vi "Configure PointScan.vi"(0 "AODAcq in":refnum<class "AODAcq.lvclass">, 3 "Recording Settings":T1, 5 "Points":i32[][](array[numeric]), 7 "GridSize":u32, 9 "Reps":u32, 11 "error in (no error)":errorcluster, 12 "Motion Points":u32, 14 "Motion Increment":u32) -> (4 "AODAcq out":refnum<class "AODAcq.lvclass">, 15 "error out":errorcluster)   [LabVIEW 2011, in "AODAcq.lvclass"]
uses:
  AODAcq.lvclass
  AODAcq.lvclass/AODAcq.ctl
  <vilib>/Utility/error.llb/Error Cluster From Error Code.vi
  Program Files/National Instruments/LabVIEW 2011/Targets/NI/FPGA/StockFPGA_IntfPrivate/ScriptTemplates/StockFPGA_PlugInRead32.vi
  <vilib>/rvi/errors/niLvFpgaAdjustHostInterfaceError.vi
  <instrlib>/niHWS/nihws.llb/niHWS Write Analog I32.vi
  <vilib>/rvi/interface/nirviReadWriteControl/nirviReadWriteControl.xnode
  FPGA_Control/AODRef.ctl
  FPGA_Control/FPGA Bitfiles/AODControl_FPGATarget_5751Acquire_F1CF9257.lvbitx
  FPGA_Control/AOD Control (FPGA).vi
  NiFpgaLv.dll
  <vilib>/FPGAPlugInAG/PXIe-7965R/niLvFpga_Read32_PXIe-7965R.vi
  <vilib>/rvi/interface/nirviReadWriteControl/niFpgaRWControlAccessTimeoutTemplate.vi
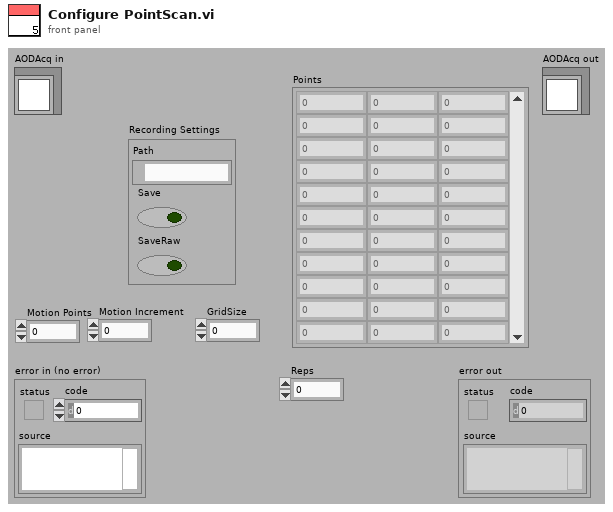
[diagram p1: front panel]
types:
  T1 = cluster{"Path":path, "Save":bool, "SaveRaw":bool}
  T2 = typedef "AODRef.ctl" = refnum<k20>
  T3 = cluster{"file handle out":u32, "ImData":u32[], "TemporalData":u32[], "MotionData":u32[], "stream reference":u32, "Open":bool, "RecordRaw":bool}
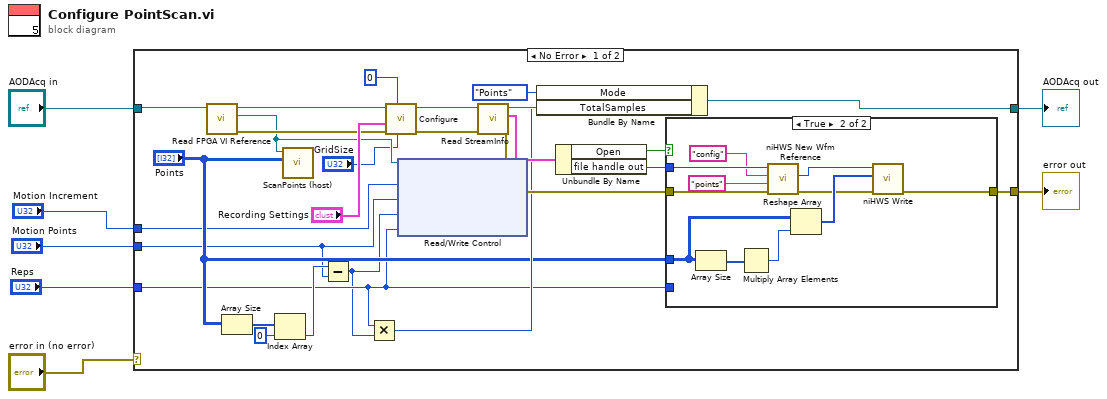
[diagram p0: block diagram]
diagram:
  n1 = case shown="No Error" "error in (no error)" {
    selector: "error in (no error)" -> [_ w47]
    tunnel: [w22 w47] -> w6
    tunnel: [w18 w46] -> w4
    tunnel: "AODAcq in" -> [w31 w46]
    tunnel: "Motion Increment" -> [w13 _]
    tunnel: "Motion Points" -> [w11 _]
    tunnel: "Reps" -> [w10 _]
    frame No Error {
      n2 = call-dynamic "Read FPGA VI Reference.vi"("AODAcq in"=w31) -> ("error out"=w28:errorcluster, "FPGA VI Reference"=w14:T2, "AODAcq out"=w30:refnum<class "AODAcq.lvclass">)  [unwired: 8 in]
      n3 = Array Size(array="Points") -> (size(s)=w21:i32[])
      n4 = Index Array(array=w21, index=0) -> (element=w12:i32)
      n5 = call "ScanPoints (host).vi"("Points"="Points", "FPGA VI Reference Out"=w14) -> ()  [unwired: 10 in]
      n6 = Subtract(x=w12, y=w11) -> (x-y=w9:u32)
      n7 = Multiply(x=w10, y=w9) -> (x*y=w17:u32)
      n8 = call-dynamic "Configure.vi"("GridSize"="GridSize", "Mode"=u32 0, "error in (no error)"=w28, "Recording Settings"="Recording Settings", "AODAcq in"=w30) -> ("error out"=w27:errorcluster, "AODAcq out"=w29:refnum<class "AODAcq.lvclass">)  [unwired: 5 in]
      n9 = xnode "Read/Write Control"("FPGA VI Reference In"=w14, "Scan.Motion Increment"=w13, "Scan.NumMotionPoints"=w11, "Scan.NumPoints"=w9, "Scan.NumReps"=w10) -> ()  [unwired: 1 in, 2 out]
      n10 = call-dynamic "Read StreamInfo.vi"("error in (no error)"=w27, "AODAcq in"=w29) -> ("error out"=w23:errorcluster, "StreamInfo"=w26:T3, "AODAcq out"=w19:refnum<class "AODAcq.lvclass">)  [unwired: 7 in]
      n11 = Bundle By Name(cluster=w19, "Mode"=enum16{"Idle", "Points", "Volume"}."Points", "TotalSamples"=w17) -> (w18:refnum<class "AODAcq.lvclass">)
      n12 = Unbundle By Name(w26) -> ("Open"=w25:bool, "file handle out"=w24:u32)
      n13 = case shown="True" w25 {
        tunnel: w24 -> [_ w40]
        tunnel: "Points" -> [_ w39]
        tunnel: w23 -> [w34 w37]
        tunnel: [w34 w35] -> w22
        tunnel: w10 -> [_ _]
        frame False {
        }
        frame True {
          n14 = Array Size(array=w39) -> (size(s)=w42:i32[])
          n15 = Multiply Array Elements(1:w42) -> (0:w43:i32)
          n16 = call <instrlib>:"niHWS New Wfm Reference.vi"("error in (no error)"=w37, "waveform name (empty)"="points", "group name (empty)"="config", "file handle in"=w40) -> ("error out"=w36:errorcluster, "waveform reference"=w45:u32)  [unwired: 5 in, 1 out]
          n17 = Reshape Array(w39, w43) -> (w44:i32[])
          n18 = call-poly <instrlib>:"niHWS Write.vi"("error in (no error)"=w36, "data"=w44, "waveform reference in"=w45) -> ("error out"=w35:errorcluster)  [unwired: 7 in, 1 out]
        }
      }
    }
    frame Error {
    }
  }
  "error out" <- w6
  "AODAcq out" <- w4
